vi "WPI_GyroXRS450_SPI_GetAngle_Optimized.vi"(6 "Reset?":bool, 8 "error in":errorcluster, 11 "GyroDevRef":T1={"DevStatus"={"status"=FALSE, "code"=0, "source"=""}, "Analog Channel"=enum."AI 0", "Gain (VoltsPerDegree/Second)"=0.0, "Gyro Type"=enum."Analog", "Handle"=0, "SPI Bus"=enum."Invalid", "Device Found"=FALSE, "Sample Rate"=1.0, "Calibrate On Open"=FALSE, "Offset"=0.0} {"Sample Rate" min=0.25 max=100.0 step=0.25}) -> (0 "error out":errorcluster, 1 "Angular Rate":dbl, 2 "Angle":dbl, 3 "GyroDevRef":T1={"DevStatus"={"status"=FALSE, "code"=0, "source"=""}, "Analog Channel"=enum."AI 0", "Gain (VoltsPerDegree/Second)"=0.0, "Gyro Type"=enum."Analog", "Handle"=0, "SPI Bus"=enum."Invalid", "Device Found"=FALSE, "Sample Rate"=1.0, "Calibrate On Open"=FALSE, "Offset"=0.0} {"Sample Rate" min=0.25 max=100.0 step=0.25})   [LabVIEW 2019]
doc: "Returns the angle, in degrees from the original heading, that the robot is currently facing.\n\nThis software is licensed. Open the labview\\readme\\WPI Robotics Library Open Source License.txt file for more information."
uses:
  <vilib>/Rock Robotics/WPI/Gyro/WPI_GyroDevRef.ctl
  <vilib>/Rock Robotics/SystemInterfaces/AI/FPGA_AIChannel.ctl
  <vilib>/Rock Robotics/SystemInterfaces/spilib/spi_bus.ctl
panel:
  out "Data Ok?":bool
  # "Analog"
  # "XRS"
  # "Analog"
  # "XRS"
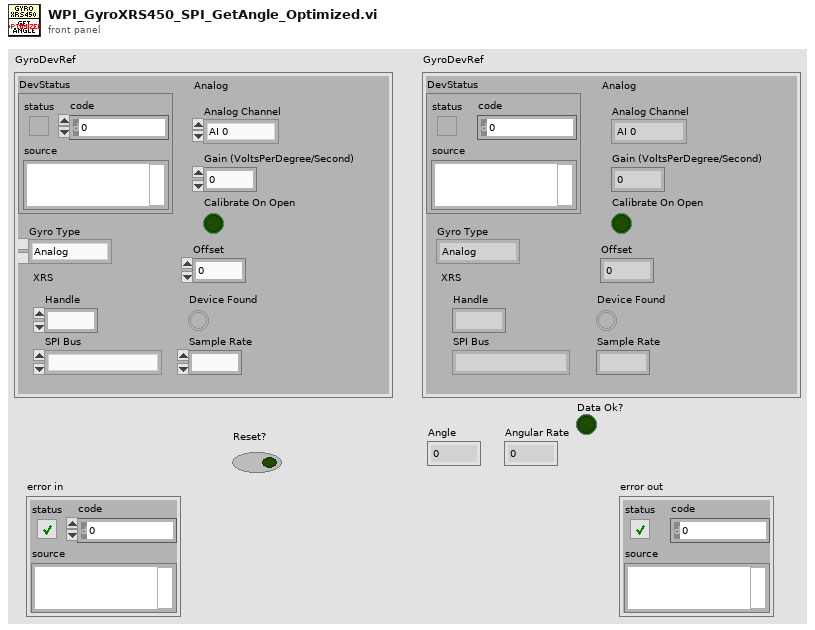
[diagram p1: front panel]
types:
  T1 = typedef "WPI_GyroDevRef.ctl" = cluster{"DevStatus":errorcluster, "Analog Channel":T2, "Gain (VoltsPerDegree/Second)":dbl, "Gyro Type":enum16{"Analog", "XRS450"}, "Handle":i32, "SPI Bus":T3, "Device Found":bool, "Sample Rate":dbl, "Calibrate On Open":bool, "Offset":dbl}
  T2 = typedef "FPGA_AIChannel.ctl" = enum8{"AI 0", "AI 1", "AI 2", "AI 3", "AI MXP 0", "AI MXP 1", "AI MXP 2", "AI MXP 3", "Invalid"}
  T3 = typedef "spi_bus.ctl" = enum16{"SPI On-Board, CS0", "SPI On-Board, CS1", "SPI On-Board, CS2", "SPI On-Board, CS3", "SPI MXP", "Invalid"}
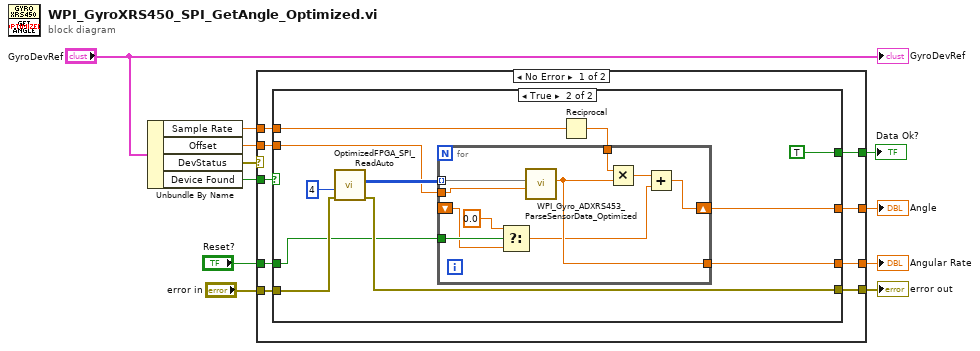
[diagram p0: block diagram]
diagram:
  n1 = Unbundle By Name("GyroDevRef") -> ("Sample Rate"=w11:dbl, "Offset"=w8:dbl, "DevStatus"=w4:errorcluster, "Device Found"=w3:bool)
  n2 = case shown="No Error" w4 {
    selector: w4 -> [_ w43]
    tunnel: w11 -> [w20 _]
    tunnel: [w19 _] -> w9
    tunnel: w8 -> [w18 _]
    tunnel: [w17 _] -> w7
    tunnel: "error in" -> [w16 _]
    tunnel: [w15 w43] -> w5
    tunnel: w3 -> [w14 _]
    tunnel: [w13 _] -> w2
    tunnel: "Reset?" -> [w12 _]
    frame No Error {
      n3 = case shown="True" w14 {
        tunnel: w20 -> [_ w25]
        tunnel: [_ w30] -> w19
        tunnel: w18 -> [_ w29]
        tunnel: [_ w28] -> w17
        tunnel: w16 -> [w21 w27]
        tunnel: [w21 w26] -> w15
        tunnel: [_ TRUE] -> w13
        tunnel: w12 -> [_ w22]
        frame False {
        }
        frame True {
          n4 = call "OptimizedFPGA_SPI_ReadAuto.vi"("error in (no error)"=w27, "Bytes per Sample"=u32 4) -> ("error out"=w26:errorcluster, "Data"=w32:u8[][])  [unwired: 8 in]
          n5 = Reciprocal(x=w25) -> (1/x=w24:dbl)
          n6 = for {
            tunnel: w32 -> [w42] mode=indexing
            tunnel: w29 -> [w41]
            shift-right: [w37] -> w28
            shift-left: _ -> [w34]
            tunnel: w24 -> [w38]
            tunnel: [w40] -> w30
            tunnel: w22 -> [w36]
            # "Offset Calibration"
            n7 = Select(t=0.0, s=w36, f=w34) -> (s? t:f=w35:dbl)
            n8 = call "WPI_Gyro_ADXRS453_ParseSensorData_Optimized.vi"("Offset"=w41, "Data"=w42) -> ("Angular Rate (deg/sec)"=w40:dbl)  [unwired: 7 in, 2 out]
            n9 = Multiply(x=w38, y=w40) -> (x*y=w39:dbl)
            n10 = Add(x=w39, y=w35) -> (x+y=w37:dbl)
          }
        }
      }
    }
    frame Error {
    }
  }
  "Angle" <- w7
  "error out" <- w5
  "Angular Rate" <- w9
  "Data Ok?" <- w2
  "GyroDevRef" <- "GyroDevRef"
